vi "LblTgl.vi"(1 "TabControl in":refnum<vi>, 8 "Numeric":i32) -> (15 "error out":errorcluster)   [LabVIEW 2014]
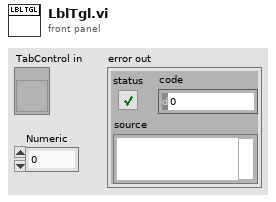
[diagram p1: front panel]
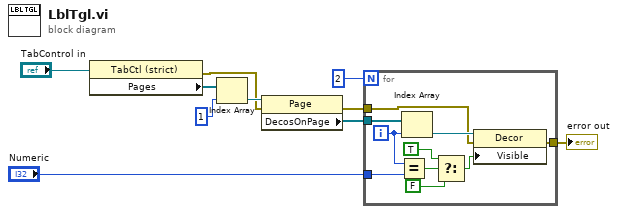
[diagram p0: block diagram]
diagram:
  n1 = property class="TabCtl (strict)"(reference="TabControl in") -> (error out=w3:errorcluster, "Pages"=w5:refnum<vi>[])  [unwired: 1 in, 1 out]
  n2 = Index Array(array=w5, index=1) -> (element=w7:refnum<vi>)
  n3 = property class="Page"(reference=w7, error in=w3) -> (error out=w2:errorcluster, "DecosOnPage"=w9:refnum<vi>[])  [unwired: 1 out]
  n4 = for {
    N: 2 -> [_]
    tunnel: w9 -> [w20]
    tunnel: "Numeric" -> [w19]
    tunnel: w2 -> [w12]
    tunnel: [w11] -> w1
    i -> [w18]
    n5 = Equal?(x=w18, y=w19) -> (x = y?=w17:bool)
    n6 = Index Array(array=w20, index=w18) -> (element=w13:refnum<vi>)
    n7 = Select(t=TRUE, s=w17, f=FALSE) -> (s? t:f=w16:bool)
    n8 = property class="Decor"(reference=w13, error in=w12, "Visible"=w16) -> (error out=w11:errorcluster)  [unwired: 1 out]
  }
  "error out" <- w1
